vi "G-String.vi"() -> (0 "SHARP":bool, 1 "TUNED":bool, 2 "FLAT":bool, 6 "FREQ at maximum":dbl, 7 "Standard FREQ":dbl)   [LabVIEW 2018]
uses:
  <vilib>/express/express analysis/Spectral/Block/exnSpectralBlock spectral measurements RMS poly.vi
  <vilib>/express/express analysis/Spectral/Block/exnSpectralBlock spectral measurements RMS DDT.vi
  <vilib>/express/express analysis/Spectral/XNode/ExpressSpectralMeasurementsBlockNode.xnode
panel:
  out "String":string
  out "FFT RMS 2":dynamicdata(graph)
  out "FFT RMS":dynamicdata(graph)
  out "Waveform Graph 2":dynamicdata(graph)
  out "Waveform Graph":dynamicdata(graph)
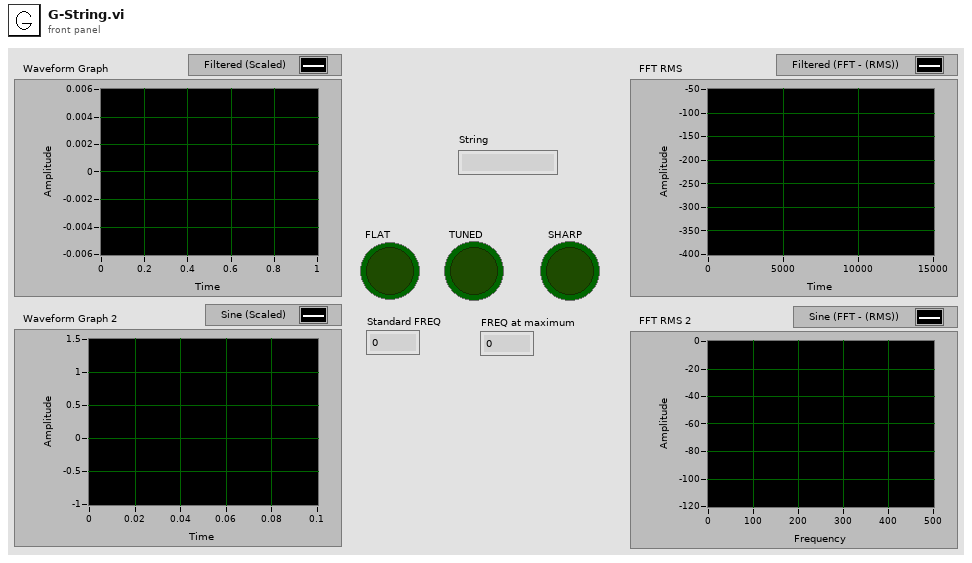
[diagram p1: front panel]
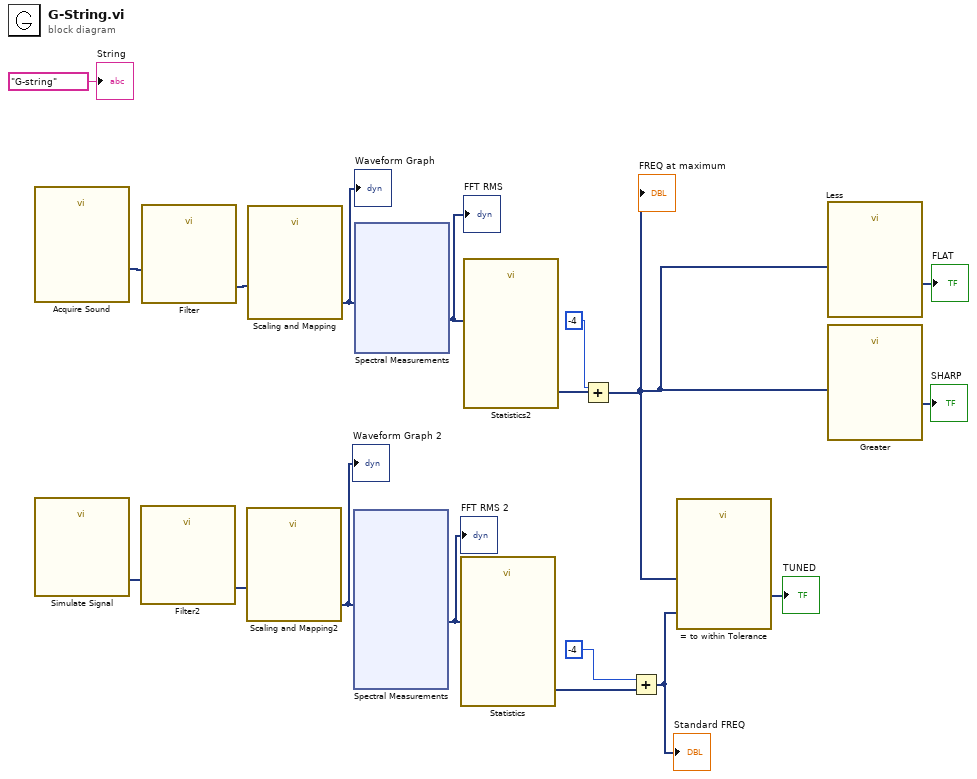
[diagram p0: block diagram]
diagram:
  n1 = call "Acquire Sound"() -> ("Data"=w16:dynamicdata)  [unwired: 18 in, 1 out]
  n2 = call "Simulate Signal"() -> ("Sine"=w15:dynamicdata)  [unwired: 14 in, 1 out]
  n3 = call "Filter2"("Signal"=w15) -> ("Filtered Signal"=w14:dynamicdata)  [unwired: 9 in, 1 out]
  n4 = call "Filter"("Signal"=w16) -> ("Filtered Signal"=w17:dynamicdata)  [unwired: 9 in, 1 out]
  n5 = call "Scaling and Mapping2"("Signals"=w14) -> ("Scaled Signals"=w18:dynamicdata)  [unwired: 9 in, 1 out]
  "Waveform Graph 2" <- w18
  n6 = call "Scaling and Mapping"("Signals"=w17) -> ("Scaled Signals"=w13:dynamicdata)  [unwired: 9 in, 1 out]
  "Waveform Graph" <- w13
  n7 = xnode "Spectral Measurements"("Signals"=w18) -> ("FFT - (RMS)"=w12:dynamicdata)  [unwired: 1 in, 2 out]
  "FFT RMS 2" <- w12
  n8 = xnode "Spectral Measurements"("Signals"=w13) -> ("FFT - (RMS)"=w11:dynamicdata)  [unwired: 1 in, 2 out]
  "FFT RMS" <- w11
  n9 = call "Statistics"("Signals"=w12) -> ("Time of Maximum"=w5:dynamicdata)  [unwired: 24 in, 2 out]
  n10 = call "Statistics2"("Signals"=w11) -> ("Time of Maximum"=w3:dynamicdata)  [unwired: 24 in, 2 out]
  n11 = Add(x=-4, y=w3) -> (x+y=w2:dynamicdata)
  "FREQ at maximum" <- w2
  n12 = Add(x=-4, y=w5) -> (x+y=w1:dynamicdata)
  "Standard FREQ" <- w1
  n13 = call "= to within Tolerance"("Operand 2"=w1, "Operand 1"=w2) -> ("Result"=→"TUNED":dynamicdata)  [unwired: 8 in, 1 out]
  n14 = call "Less"("Operand 1"=w2) -> ("Result"=→"FLAT":dynamicdata)  [unwired: 9 in, 1 out]
  n15 = call "Greater"("Operand 1"=w2) -> ("Result"=→"SHARP":dynamicdata)  [unwired: 9 in, 1 out]
  "String" <- "G-string"
